vi "DAQ Control.vi"(2 "error in":errorcluster, 3 "Control":u16, 4 "task in":refnum<k21>) -> (0 "error out":errorcluster, 1 "task out":refnum<k21>)   [LabVIEW 2023]
uses:
  <vilib>/DAQmx/write.llb/DAQmx Write (Digital Bool 1Line 1Point).vi
  <vilib>/DAQmx/miscellaneous.llb/DAQmx Fill In Error Info.vi
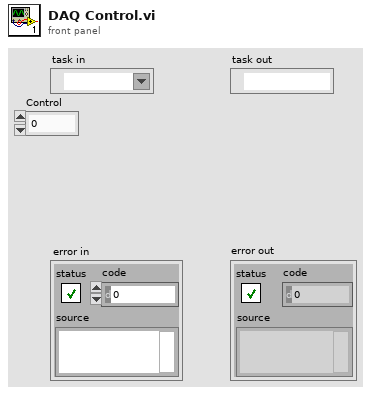
[diagram p1: front panel]
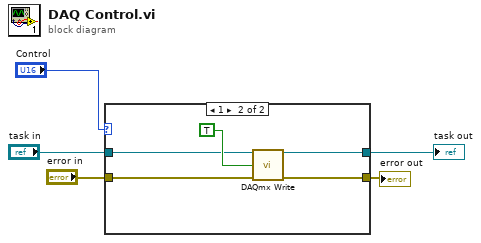
[diagram p0: block diagram]
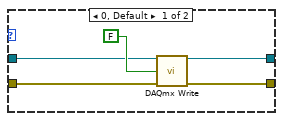
[diagram p2: hidden frame]
diagram:
  n1 = case shown="1" "Control" {
    tunnel: "error in" -> [w6 w12]
    tunnel: [w8 w14] -> w4
    tunnel: [w9 w13] -> w3
    tunnel: "task in" -> [w7 w11]
    frame 0, Default {
      n2 = call-poly <vilib>:"DAQmx Write.vi"("task/channels in"=w7, "data"=FALSE, "error in"=w6) -> ("task out"=w9:refnum<k21>, "error out"=w8:errorcluster)  [unwired: 10 in, 1 out]
    }
    frame 1 {
      n3 = call-poly <vilib>:"DAQmx Write.vi"("task/channels in"=w11, "data"=TRUE, "error in"=w12) -> ("task out"=w13:refnum<k21>, "error out"=w14:errorcluster)  [unwired: 10 in, 1 out]
    }
  }
  "error out" <- w4
  "task out" <- w3
